vi "Destination Port and IP.vi"(8 "error in (no error)":errorcluster, 11 "TCP Writer in":refnum<class "TCP Writer.lvclass">) -> (0 "error out":errorcluster, 1 "Destination Port":u16, 2 "Destination IP":string, 3 "TCP Writer out":refnum<class "TCP Writer.lvclass">)   [LabVIEW 2026, in "TALOS.lvlib" / "TCP Writer.lvlib" / "TCP Writer.lvclass"]
uses:
  TCP Writer.lvclass
  C:/LabVIEW Code/TALOS/talos/Ancestor/Ancestor/Ancestor.lvclass
  Ancestor/Ancestor/Ancestor.lvclass/Ancestor.ctl
  <vilib>/AdvancedString/Delimited String to 1D String Array (string).vi
  <vilib>/Utility/error.llb/Trim Whitespace (string).vi
  7b5259c0-7cbc-456c-8072-82aa188f7323.vi
  0e551166-5b44-4645-b46d-81060d8fbd53.vi
  d894c442-ed90-4d0b-af48-f9a51705bfb9.vi
  Ancestor/Ancestor/Read ID.vi
  Support VIs/Circus Config Param - Core.vi
  <vilib>/Utility/error.llb/Trim Whitespace One-Sided.vi
  0e551166-5b44-4645-b46d-81060d8fbd53.vi/d4db2432-cc9c-482c-8957-dac855435ef6.vi
  0e551166-5b44-4645-b46d-81060d8fbd53.vi/86fbf154-bd7b-49a2-8ab2-a837b2a95f24.vi
  0e551166-5b44-4645-b46d-81060d8fbd53.vi/3b95b01e-1ec2-4565-bcd9-7606a5281010.vi
  0e551166-5b44-4645-b46d-81060d8fbd53.vi/96a08935-737a-44b2-979c-a81d56408f7e.vi
  d894c442-ed90-4d0b-af48-f9a51705bfb9.vi/d4db2432-cc9c-482c-8957-dac855435ef6.vi
  d894c442-ed90-4d0b-af48-f9a51705bfb9.vi/86fbf154-bd7b-49a2-8ab2-a837b2a95f24.vi
  d894c442-ed90-4d0b-af48-f9a51705bfb9.vi/3b95b01e-1ec2-4565-bcd9-7606a5281010.vi
  d894c442-ed90-4d0b-af48-f9a51705bfb9.vi/96a08935-737a-44b2-979c-a81d56408f7e.vi
  Support VIs/Generate Error.vi
  Support VIs/Circus Root Path.vi
  Support VIs/TALOS Config Param.vi
  0e551166-5b44-4645-b46d-81060d8fbd53.vi/d4db2432-cc9c-482c-8957-dac855435ef6.vi/6eaecd13-6e48-4772-a921-b51ebdf84d88.vi
  0e551166-5b44-4645-b46d-81060d8fbd53.vi/d4db2432-cc9c-482c-8957-dac855435ef6.vi/d2d5f2b7-06f4-47f6-971c-049c3fdbb653.vi
  0e551166-5b44-4645-b46d-81060d8fbd53.vi/3b95b01e-1ec2-4565-bcd9-7606a5281010.vi/6eaecd13-6e48-4772-a921-b51ebdf84d88.vi
  0e551166-5b44-4645-b46d-81060d8fbd53.vi/3b95b01e-1ec2-4565-bcd9-7606a5281010.vi/d2d5f2b7-06f4-47f6-971c-049c3fdbb653.vi
  0e551166-5b44-4645-b46d-81060d8fbd53.vi/96a08935-737a-44b2-979c-a81d56408f7e.vi/6eaecd13-6e48-4772-a921-b51ebdf84d88.vi
  0e551166-5b44-4645-b46d-81060d8fbd53.vi/96a08935-737a-44b2-979c-a81d56408f7e.vi/d2d5f2b7-06f4-47f6-971c-049c3fdbb653.vi
  d894c442-ed90-4d0b-af48-f9a51705bfb9.vi/d4db2432-cc9c-482c-8957-dac855435ef6.vi/6eaecd13-6e48-4772-a921-b51ebdf84d88.vi
  d894c442-ed90-4d0b-af48-f9a51705bfb9.vi/d4db2432-cc9c-482c-8957-dac855435ef6.vi/d2d5f2b7-06f4-47f6-971c-049c3fdbb653.vi
  d894c442-ed90-4d0b-af48-f9a51705bfb9.vi/3b95b01e-1ec2-4565-bcd9-7606a5281010.vi/6eaecd13-6e48-4772-a921-b51ebdf84d88.vi
  d894c442-ed90-4d0b-af48-f9a51705bfb9.vi/3b95b01e-1ec2-4565-bcd9-7606a5281010.vi/d2d5f2b7-06f4-47f6-971c-049c3fdbb653.vi
  d894c442-ed90-4d0b-af48-f9a51705bfb9.vi/96a08935-737a-44b2-979c-a81d56408f7e.vi/6eaecd13-6e48-4772-a921-b51ebdf84d88.vi
  d894c442-ed90-4d0b-af48-f9a51705bfb9.vi/96a08935-737a-44b2-979c-a81d56408f7e.vi/d2d5f2b7-06f4-47f6-971c-049c3fdbb653.vi
  FGV/Error Memory/Get Error Description.vi
  Support VIs/Get PC name.vi
  Support VIs/Get Class Name.vi
  <vilib>/Utility/error.llb/Clear Errors.vi
  FGV/Error Memory/Error Memory Core.vi
  FGV/Error Memory/Error Crt Lvl checker.vi
  FGV/Error Memory/Error Memory Core.vi/40c8088d-b597-4017-91af-faa98e00292e.vi
  FGV/Error Memory/Error Memory Core.vi/d4a3ab98-063c-4e44-b43d-fbdcfe6c2be2.vi
  Support VIs/Global Constants.vi
  Support VIs/Global Memory.vi
  <vilib>/Utility/LVClass/Get LV Class Name.vi
  Support VIs/Is in Packed Library.vi
  Support VIs/TALOS Root path.vi
  Support VIs/Read CSV worksheet.vi
  <vilib>/Utility/error.llb/General Error Handler.vi
  <vilib>/Utility/config.llb/Open Config Data.vi
  <vilib>/Utility/config.llb/Get Section Names.vi
  <vilib>/Utility/config.llb/Get Key Names.vi
  <vilib>/Utility/config.llb/Read Key.vi
  <vilib>/Utility/config.llb/Read Key (String).vi
  <vilib>/Utility/config.llb/Close Config Data.vi
  Ancestor/Ancestor/Ancestor.lvclass
  <vilib>/Comparison/Equal/Equal Functor/Equal Functor.lvclass
  <vilib>/Comparison/Less/Less Functor/Less Functor.lvclass
  TALOS.lvlib
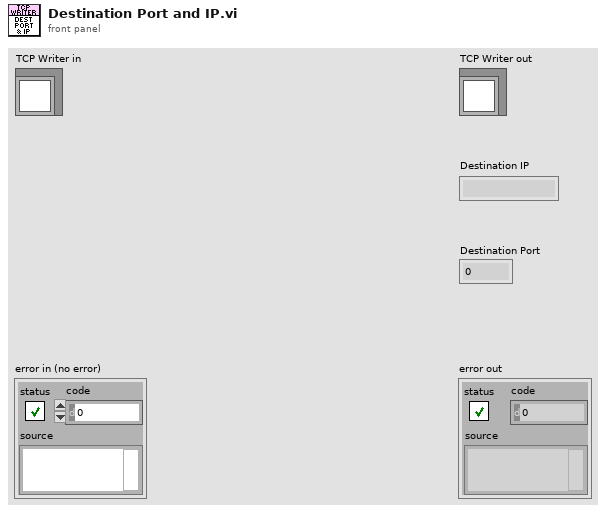
[diagram p1: front panel]
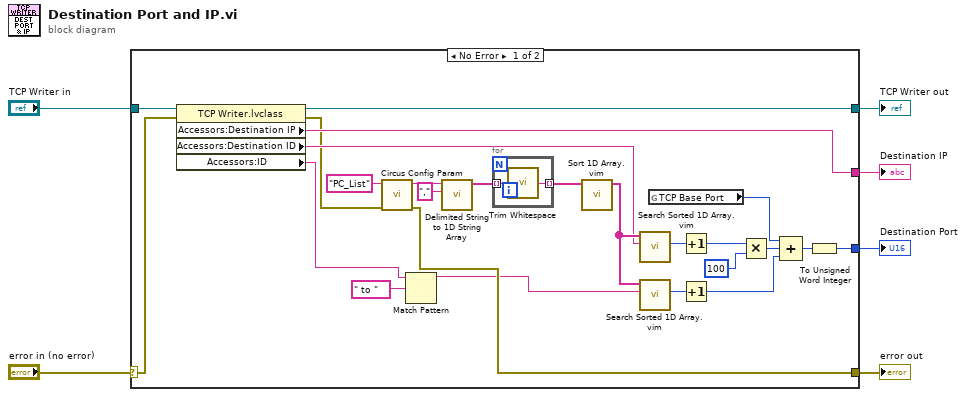
[diagram p0: block diagram]
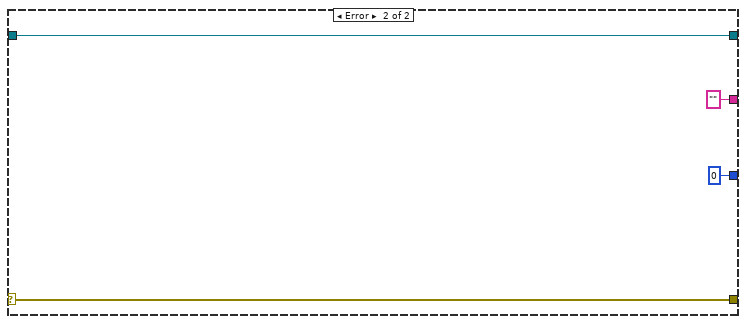
[diagram p2: hidden frame]
diagram:
  n1 = case shown="No Error" "error in (no error)" {
    selector: "error in (no error)" -> [w28 w37]
    tunnel: [w31 w37] -> w5
    tunnel: [w29 w36] -> w3
    tunnel: "TCP Writer in" -> [w30 w36]
    tunnel: [w27 "" ("Accessors:Destination IP")] -> w2
    tunnel: [w8 u16 0] -> w1
    frame No Error {
      n2 = property class="TCP Writer.lvclass"(reference=w30, error in=w28) -> (reference out=w29:refnum<class "TCP Writer.lvclass">, error out=w7:errorcluster, "Accessors:Destination IP"=w27:string, "Accessors:Destination ID"=w11:string, "Accessors:ID"=w10:string)
      n3 = call "Circus Config Param.vi"("error in (no error)"=w7, "Parameter Name"="PC_List") -> ("error out"=w31:errorcluster, "Value"=w24:string)  [unwired: 8 in]
      n4 = Match Pattern(string=w10, regular expression=" to " ("string")) -> (before substring=w9:string)  [unwired: 1 in, 3 out]
      n5 = call-poly <vilib>:"Delimited String to 1D String Array.vi"("delimiter"=",", "delimited string"=w24) -> ("string array"=w13:string[])  [unwired: 9 in]
      n6 = for {
        tunnel: w13 -> [w33] mode=indexing
        tunnel: [w32] -> w12 mode=indexing
        n7 = call-poly <vilib>:"Trim Whitespace.vi"("string"=w33) -> ("trimmed string"=w32:string)  [unwired: 1 in]
      }
      n8 = call "Sort 1D Array.vim"("unsorted array"=w12) -> ("sorted array"=w22:string[])  [unwired: 10 in]
      n9 = call "Search Sorted 1D Array.vim"("element"=w11, "sorted 1D array"=w22) -> ("nearest index"=w21:i32)  [unwired: 8 in, 1 out]
      n10 = call "Search Sorted 1D Array.vim"("element"=w9, "sorted 1D array"=w22) -> ("nearest index"=w20:i32)  [unwired: 8 in, 1 out]
      n11 = global read "Global Constants.vi" "TCP Base Port"() -> (w17:u16)
      n12 = Increment(x=w21) -> (x+1=w19:i32)
      n13 = Increment(x=w20) -> (x+1=w15:i32)
      n14 = Multiply(x=w19, y=u16 100) -> (x*y=w16:i32)
      n15 = Compound Arithmetic op=ADD(w17, w16, w15) -> (w14:i32)
      n16 = To Unsigned Word Integer(number=w14) -> (unsigned 16bit integer=w8:u16)
    }
    frame Error {
    }
  }
  "error out" <- w5
  "TCP Writer out" <- w3
  "Destination IP" <- w2
  "Destination Port" <- w1
